vi "Subvi_converter_Jonas_to_Craig.vi"(6 "theta6Jonas":dbl, 7 "theta1Jonas":dbl, 8 "theta5Jonas":dbl, 9 "theta4Jonas":dbl, 10 "theta3Jonas":dbl, 11 "theta2Jonas":dbl) -> (0 "theta5Craig":dbl, 1 "theta4Craig":dbl, 2 "theta3Craig":dbl, 3 "theta2Craig":dbl, 4 "theta6Craig":dbl, 5 "theta1Craig":dbl)   [LabVIEW 2017]
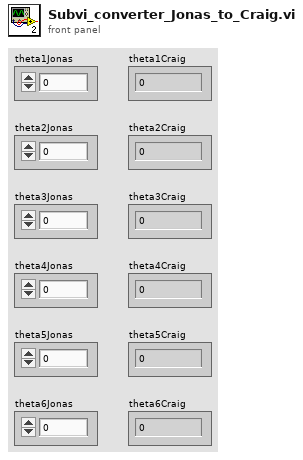
[diagram p1: front panel]
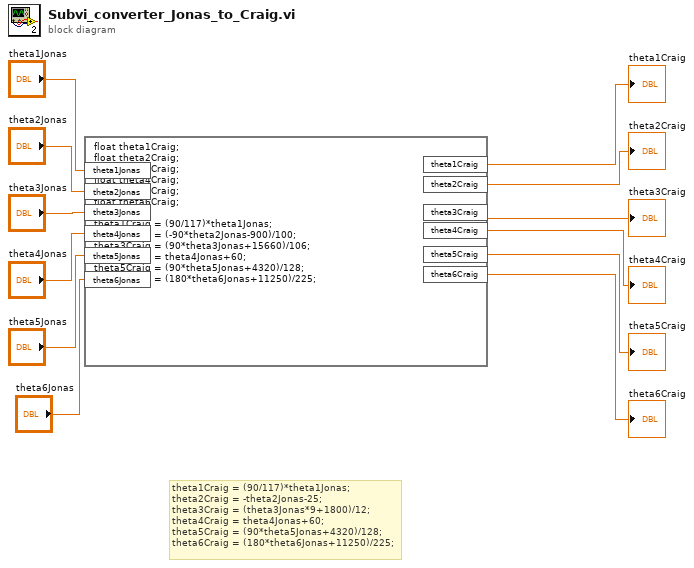
[diagram p0: block diagram]
diagram:
  # "theta1Craig = (90/117)*theta1Jonas;\ntheta2Craig = -theta2Jonas-25;\ntheta3Craig = (theta3Jonas*9+1800)/12;\ntheta4Craig = theta4Jonas+60;\ntheta5Craig = (90*theta5Jonas+4320)/128;\ntheta6Craig = (180*theta6Jonas+11250)/225;"
  n1 = formula code="float theta1Craig;\nfloat theta2Craig;\nfloat theta3Craig;\nfloat theta4Craig;\nfloat theta5Craig;\nfloat theta6Craig;\n\ntheta1Craig = (90/117)*theta1Jonas;\ntheta2Craig = (-90*theta2Jonas-900)/100;\ntheta3Craig = (90*theta3Jonas+15660)/106;\ntheta4Craig = theta4Jonas+60;\ntheta5Craig = (90*theta5Jonas+4320)/128;\ntheta6Craig = (180*theta6Jonas+11250)/225;"("theta1Jonas"="theta1Jonas", "theta3Jonas"="theta3Jonas", "theta4Jonas"="theta4Jonas", "theta5Jonas"="theta5Jonas", "theta6Jonas"="theta6Jonas", "theta2Jonas"="theta2Jonas") -> ("theta1Craig"=→"theta1Craig":dbl, "theta2Craig"=→"theta2Craig":dbl, "theta3Craig"=→"theta3Craig":dbl, "theta4Craig"=→"theta4Craig":dbl, "theta5Craig"=→"theta5Craig":dbl, "theta6Craig"=→"theta6Craig":dbl)
